vi "DSF.Engine.Execution.Framework.Set Device Ref.vi"(8 "error in (no error)":errorcluster, 10 "Device Item Ref":T1=18446744073709551615 format="%.0x", 11 "Framework in":refnum<class "DSF.Engine.Execution.Framework.lvclass">) -> (0 "error out":errorcluster, 3 "Framework out":refnum<class "DSF.Engine.Execution.Framework.lvclass">)   [LabVIEW 2016, in "DSF.Engine.lvlib" / "DSF.Engine.Execution.Framework.lvclass"]
uses:
  DSF.Engine.Execution.Framework.lvclass
  <vilib>/NI Veristand/Custom Device API/Custom Device Item Ref.ctl
  DSF.Engine.Execution.Framework.lvclass/DSF.Engine.Execution.Framework.ctl
  <vilib>/NI Veristand/Custom Device API/Custom Device API.lvlib
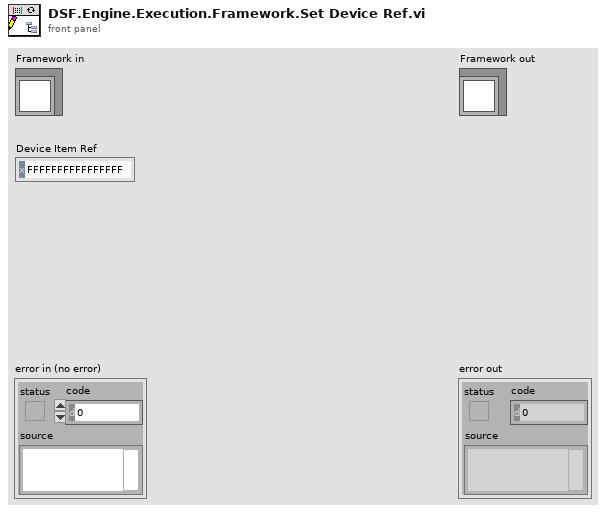
[diagram p1: front panel]
types:
  T1 = typedef "Custom Device API.lvlib/Custom Device Item Ref.ctl" = u64
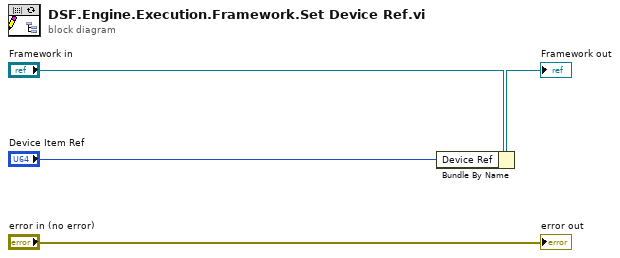
[diagram p0: block diagram]
diagram:
  n1 = Bundle By Name(cluster="Framework in", "Device Ref"="Device Item Ref") -> (→"Framework out":refnum<class "DSF.Engine.Execution.Framework.lvclass">)
  "error out" <- "error in (no error)"
